vi "to UINT16.vi"(8 "error in":errorcluster, 11 "byte":u8[](array[numeric]) format="%b") -> (0 "error out":errorcluster, 3 "UINT16":u16)   [LabVIEW 2020, in "wamplv.lvlib" / "MessagePack.lvclass"]
uses:
  MessagePack.lvclass
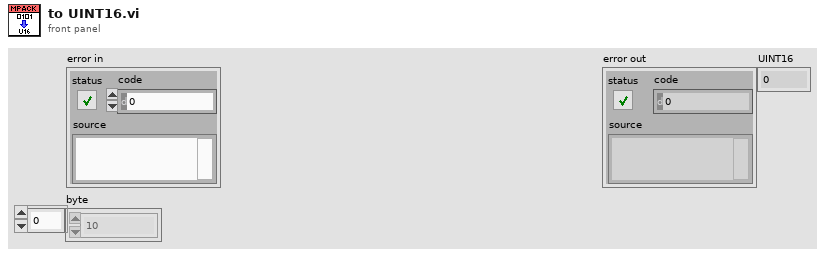
[diagram p1: front panel]
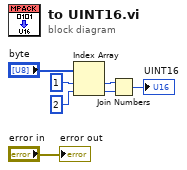
[diagram p0: block diagram]
diagram:
  n1 = Index Array(array="byte", index #1=1 ("index"), index #2=2 ("index")) -> (element #1=w3:u8, element #2=w2:u8)
  n2 = Join Numbers(hi=w3, lo=w2) -> ((hi.lo)=→"UINT16":u16)
  "error out" <- "error in"
